vi "TCP send to server.vi"(8 "error in (no error)":errorcluster, 9 "Packed In":T1, 10 "Port":u16=6341, 11 "Machine":string="localhost") -> (0 "error out":errorcluster, 1 "success":bool)   [LabVIEW 2015]
uses:
  packed var.ctl
panel:
  out "length":i32
  out "data string":string
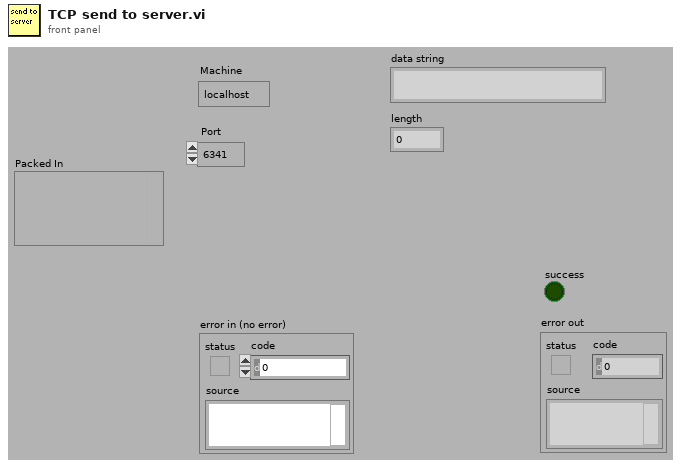
[diagram p1: front panel]
types:
  T1 = typedef "packed var.ctl" = variant
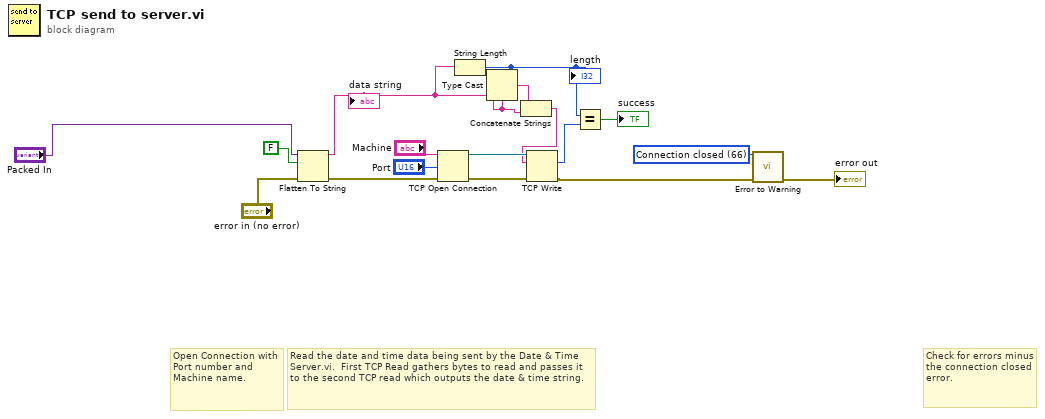
[diagram p0: block diagram]
diagram:
  w15 = 66 items=["No Error", "Argument Error", "Memory Full", "Out of Zone", "End of File", "File Already Open", "Generic File IO Error", "File Not Found", "File Permission Error", "Disk Full", "Duplicate Path", "Too Many Files Open", "Not Enabled", "Resource File Not Found", "Cannot Add Resource", "Resource Not Found", "Image Not Found", "Image Memory Error", "Pen Does Not Exist", "Config Bad Type", "Config Token Not Found", "Config Parse Error", "Config Memory Error", "Bad External Code Format", "Bad External Code Offset", "External Code Not Present", "Null Window", "Destroy Window Mixup", "Null Menu", "Print Aborted", "Bad Print Record", "Print Driver Error", "Windows Error During Print", "Memory Error During Print", "Print Dialog Error", "Generic Print Error", "Invalid Device Refnum", "Device Not Found", "Device Parameter Error", "Device Unit Error", "Can't Open Device", "Device Call Aborted", "Generic Error", "Cancelled By User", "Object ID Too Low", "Object ID Too High", "Object Not In Heap", "Unknown Heap", "Bad DefProc ID", "DefProc Not In Table", "Message Out Of Range", "Null Method", "Unknown Message", "Manager Call Not Supported", "Bad address", "Connection In progress", "Connection timed out", "Connection is already in progress", "Network attribute not supported", "Network error", "Address in use", "System out of memory", "Connection aborted", "Connection refused", "Connection is not connected", "Connection is already connected", "Connection closed", "Initialize error (interapplication manager)", "Bad occurrence", "Wait on unbound occurrence handler", "Occurrence queue overflow", "Bad path", "Semaphore not signaled", "Unrecognized type (interapplication manager)"] ("1st Error to Convert")
  # "Check for errors minus the connection closed error."
  # "Read the date and time data being sent by the Date & Time Server.vi.  First TCP Read gathers bytes to read and passes it to the second TCP read which outputs the date & time string."
  # "Open Connection with Port number and Machine name."
  n1 = Flatten To String(anything="Packed In", prepend array or string size? (T)=FALSE, error in (no error)="error in (no error)") -> (data string=w4:string, error out=w11:errorcluster)  [unwired: 1 in, 1 out]
  "data string" <- w4
  n2 = TCP Open Connection(address="Machine", remote port or service name="Port", error in (no error)=w11) -> (connection ID=w13:refnum<k5>, error out=w12:errorcluster)  [unwired: 2 in]
  n3 = String Length(string=w4) -> (length=w6:i32)
  "length" <- w6
  n4 = Type Cast(type=w4, x=w6) -> (*(type *) &x=w5:string)
  n5 = Concatenate Strings(w5, w4) -> (w3:string)
  n6 = TCP Write(connection ID=w13, data in=w3, error in (no error)=w12) -> (bytes written=w9:i32, error out=w7:errorcluster)  [unwired: 1 in, 1 out]
  n7 = Equal?(x=w6, y=w9) -> (x = y?=→"success":bool)
  n8 = call <vilib>:"Error to Warning.vi"("1st Error to Convert"=w15, "error in"=w7) -> ("warning out"=→"error out":errorcluster)  [unwired: 13 in]
